vi "PXI-Update DI.vi"(0 "DI Tasks":T1[](array[typedef]), 5 "Skip samples":i32, 11 "error in (no error)":errorcluster, 12 "cycle":i32) -> (15 "error out":errorcluster)   [LabVIEW 2020]
uses:
  Type Defs/Task Struct.ctl
  PXI Globals.vi
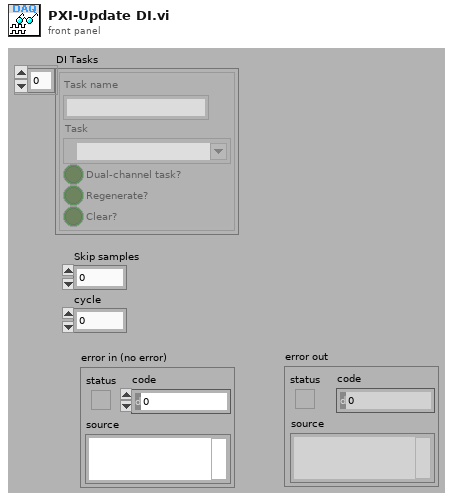
[diagram p1: front panel]
types:
  T1 = typedef "Task Struct.ctl" = cluster{"Task name":string, "Task":refnum<k21>, "Dual-channel task?":bool, "Regenerate?":bool, "Clear?":bool}
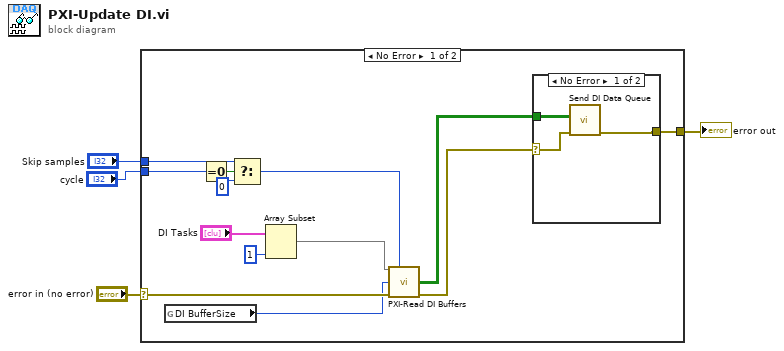
[diagram p0: block diagram]
diagram:
  n1 = case shown="No Error" "error in (no error)" {
    selector: "error in (no error)" -> [w16 w22]
    tunnel: [w17 w22] -> w4
    tunnel: "Skip samples" -> [w7 _]
    tunnel: "cycle" -> [w6 _]
    frame No Error {
      n2 = global read "PXI Globals.vi" "DI BufferSize"() -> (w12:i32)
      n3 = Equal To 0?(x=w6) -> (x = 0?=w9:bool)
      n4 = Select(t=w7, s=w9, f=0) -> (s? t:f=w5:i32)
      n5 = Array Subset(array="DI Tasks", length=1) -> (w11:T1[])  [unwired: 1 in]
      n6 = call "PXI-Read DI Buffers.vi"("DI Tasks"=w11, "Samples to skip"=w5, "Samples per channel"=w12, "error in (no error)"=w16) -> ("DI Waveforms"=w15:bool[][], "error out"=w14:errorcluster)  [unwired: 10 in]
      n7 = case shown="No Error" w14 {
        selector: w14 -> [w20 w21]
        tunnel: w15 -> [w18 _]
        tunnel: [w19 w21] -> w17
        frame No Error {
          n8 = call "Send DI Data Queue.vi"("error in"=w20, "DI Waveforms"=w18) -> ("error out"=w19:errorcluster)  [unwired: 5 in]
        }
        frame Error {
        }
      }
    }
    frame Error {
    }
  }
  "error out" <- w4
